vi "Get Matched Pairs.vi"(7 "interp. method":enum16{"nearest", "linear"}(ring)=enum."linear", 8 "Cluster 2":T1={"Colour"=0, "Inst type"=enum."Raw voltage", "Inst name"="", "Symbol"="", "Code name"="", "Extra Info"="", "Inst Array"=enum."PWA", "U"=0.0, "u^2"=0.0, "u^3"=0.0, "u^4"=0.0, "Skew_u"=0.0, "Kurt_u"=0.0, "Sd Error in Mean"=0.0, "% u'/U"=0.0, "X"=0.0, "Y"=0.0, "Z"=0.0, "Timescale integral Estimate"=0.0, "Sd Error in Variance"=0.0, "Calib File"=path "", "Calib Constants"=[], "Output Position"=FALSE, "Stats"=enum."None", "Av Sampling Rate"=0.0, "Av No of Samples"=0.0, "Total Meas Time (s)"=0.0, "OrigChName"="", "Max value"=0.0, "Min value"=0.0, "Req Sample Rate Hz"=0.0, "Sync Delay Time (s)"=0.0, "Ch No"=0, "Device"="", "Use Latest Calib"=FALSE, "Port"="", "Metadata Ch Names"=[], "Metadata Ch Values"=[], "Label"="", "chState"=enum."Solo", "Point Drift"=0.0, "inputConfig"=""} {"Kurt_u" format="%_3g"; "u^4" format="%_3g"; "u^3" format="%_3g"; "Sd Error in Variance" format="%_3g"; "u^2" format="%_3g"; "Sd Error in Mean" format="%_3g"; "U" format="%_3g"; "Sync Delay Time (s)" format="%.4f"; "Total Meas Time (s)" format="%_5g"; "Skew_u" format="%_3g"; "% u'/U" format="%_3g"}, 9 "Cluster 1":T1={"Colour"=0, "Inst type"=enum."Raw voltage", "Inst name"="", "Symbol"="", "Code name"="", "Extra Info"="", "Inst Array"=enum."PWA", "U"=0.0, "u^2"=0.0, "u^3"=0.0, "u^4"=0.0, "Skew_u"=0.0, "Kurt_u"=0.0, "Sd Error in Mean"=0.0, "% u'/U"=0.0, "X"=0.0, "Y"=0.0, "Z"=0.0, "Timescale integral Estimate"=0.0, "Sd Error in Variance"=0.0, "Calib File"=path "", "Calib Constants"=[], "Output Position"=FALSE, "Stats"=enum."None", "Av Sampling Rate"=0.0, "Av No of Samples"=0.0, "Total Meas Time (s)"=0.0, "OrigChName"="", "Max value"=0.0, "Min value"=0.0, "Req Sample Rate Hz"=0.0, "Sync Delay Time (s)"=0.0, "Ch No"=0, "Device"="", "Use Latest Calib"=FALSE, "Port"="", "Metadata Ch Names"=[], "Metadata Ch Values"=[], "Label"="", "chState"=enum."Solo", "Point Drift"=0.0, "inputConfig"=""} {"Kurt_u" format="%_3g"; "u^4" format="%_3g"; "u^3" format="%_3g"; "Sd Error in Variance" format="%_3g"; "u^2" format="%_3g"; "Sd Error in Mean" format="%_3g"; "U" format="%_3g"; "Sync Delay Time (s)" format="%.4f"; "Total Meas Time (s)" format="%_5g"; "Skew_u" format="%_3g"; "% u'/U" format="%_3g"}, 10 "Time (s) 2":dbl[](array[numeric]), 11 "Time (s) 1":dbl[](array[numeric])) -> (2 "Time Window (ms)":dbl, 3 "Cluster out":cluster{"Cluster":T5, "Cluster":T5, dbl})   [LabVIEW 2022 SP3]
uses:
  Controls/Resample mode.ctl
  Controls/Inst_type.ctl
  Controls/Instrument_Array.ctl
  Controls/Analysis_info_cluster.ctl
  Controls/channelState.ctl
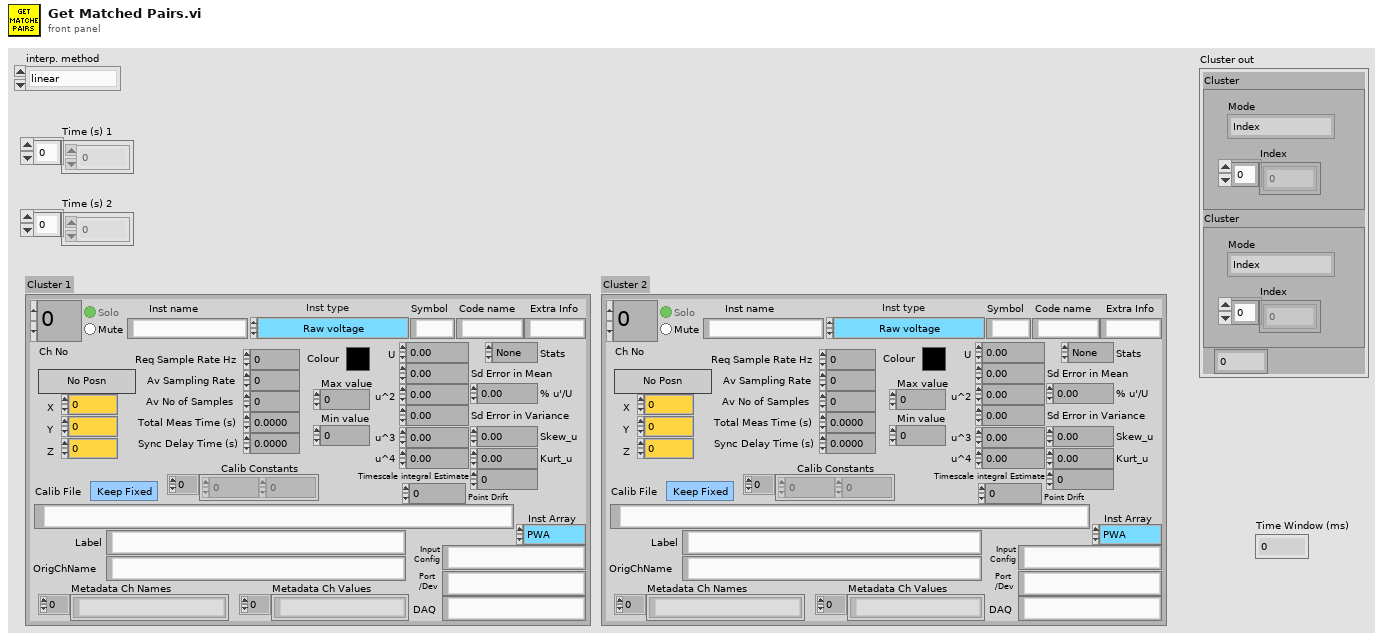
[diagram p1: front panel]
types:
  T1 = typedef "Analysis_info_cluster.ctl" = cluster{"Colour":u32, "Inst type":T2, "Inst name":string, "Symbol":string, "Code name":string, "Extra Info":string, "Inst Array":T3, "U":dbl, "u^2":dbl, "u^3":dbl, "u^4":dbl, "Skew_u":dbl, "Kurt_u":dbl, "Sd Error in Mean":dbl, "% u'/U":dbl, "X":dbl, "Y":dbl, "Z":dbl, "Timescale integral Estimate":dbl, "Sd Error in Variance":dbl, "Calib File":path, "Calib Constants":dbl[], "Output Position":bool, "Stats":enum16{"None", "Basic", "Full"}, "Av Sampling Rate":dbl, "Av No of Samples":dbl, "Total Meas Time (s)":dbl, "OrigChName":string, "Max value":dbl, "Min value":dbl, "Req Sample Rate Hz":dbl, "Sync Delay Time (s)":dbl, "Ch No":i16, "Device":string, "Use Latest Calib":bool, "Port":string, "Metadata Ch Names":string[], "Metadata Ch Values":string[], "Label":string, "chState":T4, "Point Drift":dbl, "inputConfig":string}
  T2 = typedef "Inst_type.ctl" = enum16{"Raw voltage", "Raw with zero offsetting", "Propeller anemometer", "Pressure Transducer", "Pitot-static tube", "Hot wire", "Cross wire 1", "Cross wire 2", "Generic Linear", "Generic Polynomial", "Generic BackPoly", "Fast FID", "Thermocouple", "Cold wire", "Pulsed Wire", "LDA Vel", "LDA Tran time", "LDA Arr time", "Microphone"}
  T3 = typedef "Instrument_Array.ctl" = enum16{"PWA", "LDA", "Analogue"}
  T4 = typedef "channelState.ctl" = enum32{"No Selection", "Solo", "Mute"}
  T5 = typedef "Resample mode.ctl" = cluster{"Mode":enum16{"Index", "Interpolate"}, "Index":dbl[]}
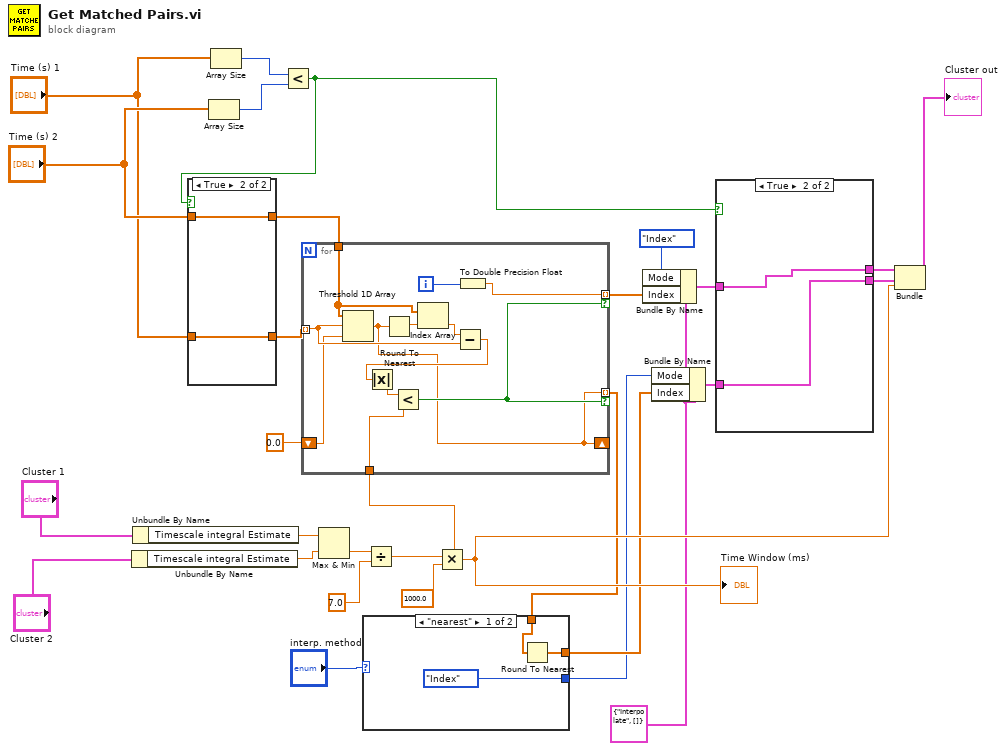
[diagram p0: block diagram]
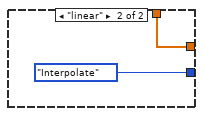
[diagram p2: hidden frame]
diagram:
  w19 = T5 {"Mode"=enum."Interpolate", "Index"=[]} ("Cluster")
  n1 = Unbundle By Name("Cluster 2") -> ("Timescale integral Estimate"=w2:dbl)
  n2 = Unbundle By Name("Cluster 1") -> ("Timescale integral Estimate"=w1:dbl)
  n3 = Array Size(array="Time (s) 2") -> (size(s)=w8:i32)
  n4 = Array Size(array="Time (s) 1") -> (size(s)=w9:i32)
  n5 = Less?(x=w9, y=w8) -> (x < y?=w12:bool)
  n6 = case shown="True" w12 {
    tunnel: "Time (s) 2" -> [w30 w33]
    tunnel: [w31 w33] -> w10
    tunnel: "Time (s) 1" -> [w31 w32]
    tunnel: [w30 w32] -> w11
    frame False {
    }
    frame True {
    }
  }
  n7 = Max & Min(x=w1, y=w2) -> (min(x,y)=w3:dbl)  [unwired: 1 out]
  n8 = Divide(x=w3, y=7.0) -> (x/y=w5:dbl)
  n9 = for {
    tunnel: w11 -> [w41] mode=indexing
    tunnel: w10 -> [w45]
    tunnel: w5 -> [w40]
    shift-right: [w35] -> _
    shift-left: 0.0 -> [w39]
    tunnel: [w35] -> w23 mode=indexing if=w38
    tunnel: [w36] -> w17 mode=indexing if=w38
    i -> [w37]
    n10 = Threshold 1D Array(1:w39, 2:w41, 3:w45) -> (0:w35:dbl)
    n11 = Round To Nearest(number=w35) -> (nearest integer value=w34:dbl)
    n12 = Index Array(array=w45, index=w34) -> (element=w43:dbl)
    n13 = Subtract(x=w43, y=w41) -> (x-y=w42:dbl)
    n14 = Absolute Value(x=w42) -> (abs(x)=w44:dbl)
    n15 = Less?(x=w44, y=w40) -> (x < y?=w38:bool)
    n16 = To Double Precision Float(number=w37) -> (double precision float=w36:dbl)
  }
  n17 = case shown="\"nearest\"" "interp. method" {
    tunnel: [enum16{"Index", "Interpolate"}."Index" ("Mode") enum16{"Index", "Interpolate"}."Interpolate" ("Mode")] -> w20
    tunnel: [w46 w49] -> w22
    tunnel: w23 -> [w47 w49]
    frame "nearest" {
      n18 = Round To Nearest(number=w47) -> (nearest integer value=w46:dbl[])
    }
    frame "linear" {
    }
  }
  n19 = Multiply(x=w5, y=1000.0) -> (x*y=w29:dbl)
  "Time Window (ms)" <- w29
  n20 = Bundle By Name(cluster=w19, "Mode"=enum16{"Index", "Interpolate"}."Index", "Index"=w17) -> (w24:T5)
  n21 = Bundle By Name(cluster=w19, "Mode"=w20, "Index"=w22) -> (w27:T5)
  n22 = case shown="True" w12 {
    tunnel: w24 -> [w52 w54]
    tunnel: [w51 w54] -> w25
    tunnel: [w52 w53] -> w26
    tunnel: w27 -> [w51 w53]
    frame False {
    }
    frame True {
    }
  }
  n23 = Bundle("Cluster"=w25, "Cluster"=w26, w29) -> (→"Cluster out":cluster{"Cluster":T5, "Cluster":T5, dbl})  [unwired: 1 in]
